vi "Config Instrument.vi"(0 "VISA resource name":refnum<visa-resource-name>, 1 "External Scanner\nMode (0: Off)":u16(ring) items=["Off", "Manual", "Autoscan", "Slave"], 2 "External Scanner\nInput (1)":dbl=1.0 min=1.0 max=16.0 step=1.0, 3 "External Scanner\nAutoscan Interval (2)":dbl=2.0 min=2.0 max=200.0 step=1.0, 5 "Remote Interface\nMode (0: Local)":u16(ring) items=["Local", "Remote", "Remote w/ Lockout"], 7 "Lock-Out (F: Lock-Out Off)":bool, 9 "Lock-Out Code (123)":dbl=123.0 min=0.0 max=999.0 step=1.0, 11 "error in (no error)":errorcluster, 12 "Beeper (F: Beeper Off)":bool) -> (4 "VISA resource name out":refnum<visa-resource-name>, 15 "error out":errorcluster)   [LabVIEW 2020, in "Lake Shore Cryotronics 340.lvlib"]
doc: "This VI configures various instrument settings. Parameters configured are;\nRemote interface mode, Keypad lock out, External scanner mode, Audible beeper status."
uses:
  Lake Shore Cryotronics 340.lvlib
panel:
  # "Lock-Out On\nLock-Out Off"
  # "Beeper On\nBeeper Off"
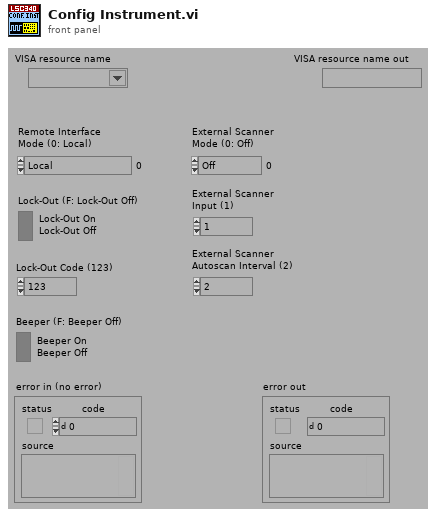
[diagram p1: front panel]
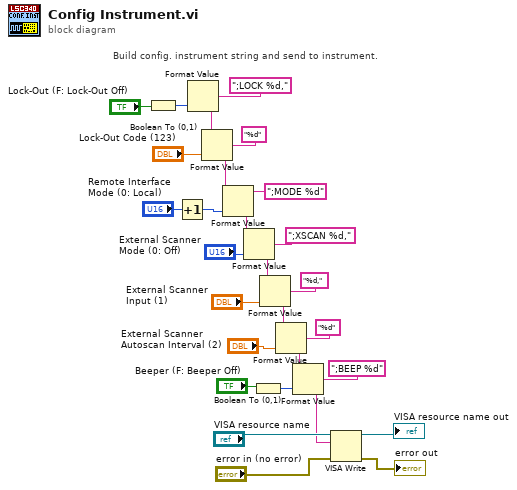
[diagram p0: block diagram]
diagram:
  # "Build config. instrument string and send to instrument."
  n1 = Boolean To (0,1)(Boolean="Lock-Out (F: Lock-Out Off)") -> (0, 1=w23:i16)
  n2 = Increment(x="Remote Interface\nMode (0: Local)") -> (x+1=w24:u16)
  n3 = Format Value(format string=";LOCK %d,", value (0)=w23) -> (output string=w20:string)  [unwired: 1 in]
  n4 = Format Value(string ("")=w20, format string="%d", value (0)="Lock-Out Code (123)") -> (output string=w1:string)
  n5 = Format Value(string ("")=w1, format string=";MODE %d", value (0)=w24) -> (output string=w2:string)
  n6 = Format Value(string ("")=w2, format string=";XSCAN %d,", value (0)="External Scanner\nMode (0: Off)") -> (output string=w16:string)
  n7 = Boolean To (0,1)(Boolean="Beeper (F: Beeper Off)") -> (0, 1=w11:i16)
  n8 = Format Value(string ("")=w16, format string="%d,", value (0)="External Scanner\nInput (1)") -> (output string=w12:string)
  n9 = Format Value(string ("")=w12, format string="%d", value (0)="External Scanner\nAutoscan Interval (2)") -> (output string=w9:string)
  n10 = Format Value(string ("")=w9, format string=";BEEP %d", value (0)=w11) -> (output string=w3:string)
  n11 = VISA Write(VISA resource name="VISA resource name", write buffer=w3, error in (no error)="error in (no error)") -> (VISA resource name out=→"VISA resource name out":refnum<visa-resource-name>, error out=→"error out":errorcluster)  [unwired: 1 out]
